vi "xiImageMng - Manager.vi"(7 "State":T3, 8 "error in (no error)":errorcluster, 11 "Properties In":T1) -> (0 "error out":errorcluster, 3 "Properties Out":T1)   [LabVIEW 2015]
doc: "Get / Set Current Image dimension. This VI is called when 1D U8 image data is converted to LabVIEW or IMAQ Image. To get image dimension in this way is much faster than calling GetImageWidth and GetImageHeight."
uses:
  xiImageMng - Attributes.ctl
  PRM/IMG_FORMAT/IMG_DATA_FORMAT.ctl
  xiImageMng - State.ctl
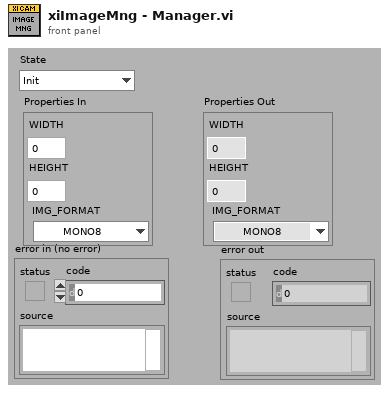
[diagram p1: front panel]
types:
  T1 = typedef "xiImageMng - Attributes.ctl" = cluster{"WIDTH":i32, "HEIGHT":i32, "IMG_FORMAT":T2}
  T2 = typedef "IMG_DATA_FORMAT.ctl" = enum16{"MONO8", "MONO16", "RGB24", "RGB32", "RGBPLANAR", "RAW8", "RAW16"}
  T3 = typedef "xiImageMng - State.ctl" = enum16{"Init", "GetProperties", "SetProperties"}
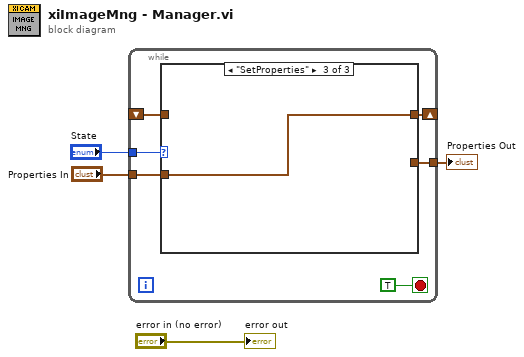
[diagram p0: block diagram]
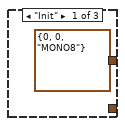
[diagram p2: hidden frame]
diagram:
  n1 = while {
    tunnel: "State" -> [w9]
    shift-right: [w8] -> _
    shift-left: _ -> [w7]
    tunnel: [w6] -> w2
    tunnel: "Properties In" -> [w5]
    stop <- TRUE stop-if-true
    n2 = case shown="\"SetProperties\"" w9 {
      tunnel: [T1 {"WIDTH"=0, "HEIGHT"=0, "IMG_FORMAT"=enum."MONO8"} ("ImageAttrib") w12 w13] -> w8
      tunnel: w7 -> [_ w12 _]
      tunnel: [_ w12 _] -> w6
      tunnel: w5 -> [_ _ w13]
      frame "Init" {
      }
      frame "GetProperties" {
      }
      frame "SetProperties" {
      }
    }
  }
  "Properties Out" <- w2
  "error out" <- "error in (no error)"
